vi "New NonOOPlayer.vi"(8 "error in":errorcluster, 11 "PlayerFilePath":path) -> (0 "error out":errorcluster, 3 "NonOOPlayer out":refnum<class "NonOOPlayer.lvclass">)   [LabVIEW 2020, in "NonOOPlayer.lvclass"]
uses:
  NonOOPlayer.lvclass
  NonOOPlayer.lvclass/NonOOPlayer.ctl
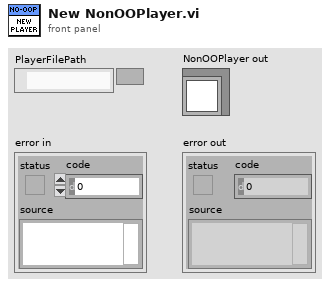
[diagram p1: front panel]
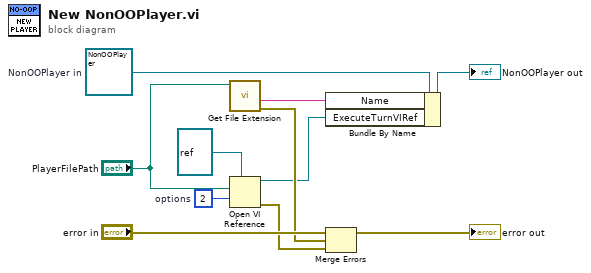
[diagram p0: block diagram]
diagram:
  w1 = 2  # options
  w5 = refnum<class "NonOOPlayer.lvclass"> refnum  # NonOOPlayer in
  n1 = call <vilib>:"Get File Extension.vi"("file"="PlayerFilePath") -> ("error out"=w8:errorcluster, "filename without extension"=w3:string)  [unwired: 6 in, 3 out]
  n2 = Open VI Reference(type specifier VI Refnum (for type only)=refnum<vi> refnum, vi path="PlayerFilePath", options=w1) -> (vi reference=w2:refnum<vi>, error out=w9:errorcluster)  [unwired: 3 in]
  n3 = Bundle By Name(cluster=w5, "Name"=w3, "ExecuteTurnVIRef"=w2) -> (→"NonOOPlayer out":refnum<class "NonOOPlayer.lvclass">)
  n4 = Merge Errors("error in", w8, w9) -> (→"error out":errorcluster)
